vi "ReversedEngineering MergeEdges.vi"(10 "ExistingEdges":refnum<class "AbstractEdge.lvclass">[](array[class]), 11 "EdgesCreated":refnum<class "AbstractEdge.lvclass">[](array[class])) -> (3 "EdgesOut":refnum<class "AbstractEdge.lvclass">[](array[class]))   [LabVIEW 2014]
uses:
  <resource>/Framework/Providers/Open_GDS/UML/AbstractEdge_class/AbstractEdge.lvclass
  <resource>/Framework/Providers/Open_GDS/UML/ClassRelationshipEdge_class/ClassRelationshipEdge.lvclass
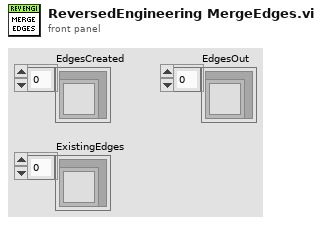
[diagram p1: front panel]
types:
  T1 = typedef "ClassRelationshipEdge.lvclass/GetAllInfoType.ctl" = cluster{"start":refnum<class "AbstractNode.lvclass">, "end":refnum<class "AbstractNode.lvclass">, "lineStyle":T2, "arrowHead":T3, "arrowHead":T3}
  T2 = typedef "LineStyle.lvclass/LineStyleType.ctl" = enum16{"SOLID", "DOTTED"}
  T3 = typedef "ArrowHead.lvclass/ArrowHeadType.ctl" = enum16{"NONE", "TRIANGLE", "BLACK_TRIANGLE", "V", "HALF_V", "DIAMOND", "BLACK_DIAMOND"}
  T4 = typedef "ClassRelationshipEdge.lvclass/PathInfoType.ctl" = cluster{"bentStyleRef":refnum<class "BentStyle.lvclass">, "startConnectionOffset":cluster{"x":i32, "y":i32}, "MidLineOffset":cluster{"x":i32, "y":i32}, "endConnectionOffset":cluster{"x":i32, "y":i32}}
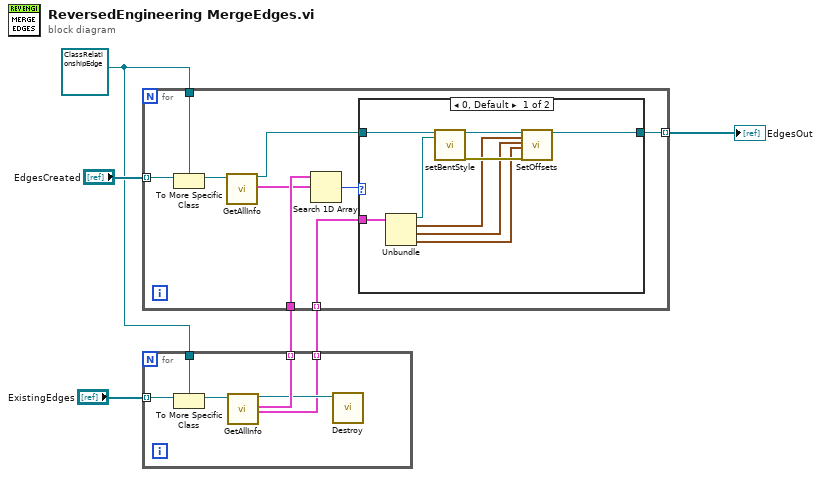
[diagram p0: block diagram]
diagram:
  w4 = refnum<class "ClassRelationshipEdge.lvclass"> refnum ("reference")
  n1 = for {
    tunnel: "ExistingEdges" -> [w12] mode=indexing
    tunnel: w4 -> [w11]
    tunnel: [w9] -> w3 mode=indexing
    tunnel: [w7] -> w1 mode=indexing
    n2 = To More Specific Class(target class=w11, reference=w12) -> (specific class reference=w10:refnum<class "ClassRelationshipEdge.lvclass">)  [unwired: 1 in, 1 out]
    n3 = call-dynamic "GetAllInfo.vi"("reference in"=w10) -> ("reference out"=w8:refnum<class "ClassRelationshipEdge.lvclass">, "AllInfo"=w9:T1, "PathInfo"=w7:T4)  [unwired: 15 in, 1 out]
    n4 = call-dynamic "Destroy.vi"("reference"=w8) -> ()  [unwired: 18 in, 1 out]
  }
  n5 = for {
    tunnel: "EdgesCreated" -> [w21] mode=indexing
    tunnel: w4 -> [w20]
    tunnel: w3 -> [w18]
    tunnel: [w14] -> w2 mode=indexing
    tunnel: w1 -> [w13] mode=indexing
    n6 = To More Specific Class(target class=w20, reference=w21) -> (specific class reference=w19:refnum<class "ClassRelationshipEdge.lvclass">)  [unwired: 1 in, 1 out]
    n7 = call-dynamic "GetAllInfo.vi"("reference in"=w19) -> ("reference out"=w15:refnum<class "ClassRelationshipEdge.lvclass">, "AllInfo"=w17:T1)  [unwired: 15 in, 2 out]
    n8 = Search 1D Array(1D array=w18, element=w17) -> (index of element=w16:i32)  [unwired: 1 in]
    n9 = case shown="0, Default" w16 {
      tunnel: w15 -> [w29 w31]
      tunnel: [w22 w31] -> w14
      tunnel: w13 -> [w30 _]
      frame 0, Default {
        n10 = Unbundle(w30) -> ("bentStyleRef"=w28:refnum<class "BentStyle.lvclass">, "startConnectionOffset"=w25:cluster{"x":i32, "y":i32}, "MidLineOffset"=w24:cluster{"x":i32, "y":i32}, "endConnectionOffset"=w23:cluster{"x":i32, "y":i32})
        n11 = call <resource>:"setBentStyle.vi"("reference"=w29, "newBentStyle"=w28) -> ("reference out"=w26:refnum<class "ClassRelationshipEdge.lvclass">, "error out"=w27:errorcluster)  [unwired: 16 in]
        n12 = call <resource>:"SetOffsets.vi"("reference"=w26, "startConnectionOffset"=w25, "MidLineOffset"=w24, "endConnectionOffset"=w23, "error in (no error)"=w27) -> ("reference out"=w22:refnum<class "ClassRelationshipEdge.lvclass">)  [unwired: 13 in, 1 out]
      }
      frame -1 {
      }
    }
  }
  "EdgesOut" <- w2
